vi "Parse TMC_Telemetry.vi"(10 "Variant":variant) -> (2 "Automated_Telemetry":T1 {"Register 1"."Spare" format="%04x"; "Register 2"."Spare" format="%04x"; "Register 4"."Spare" format="%04x"; "Register 5"."Spare" format="%04x"; "Register 6"."Spare" format="%04x"; "Register 7"."Spare" format="%04x"; "Register 8"."Spare" format="%04x"; "Register 9"."Spare" format="%.0x"; "Register 9"."A_D_Value" format="%.0x"; "Register D"."Spare" format="%03x"})   [LabVIEW 2019]
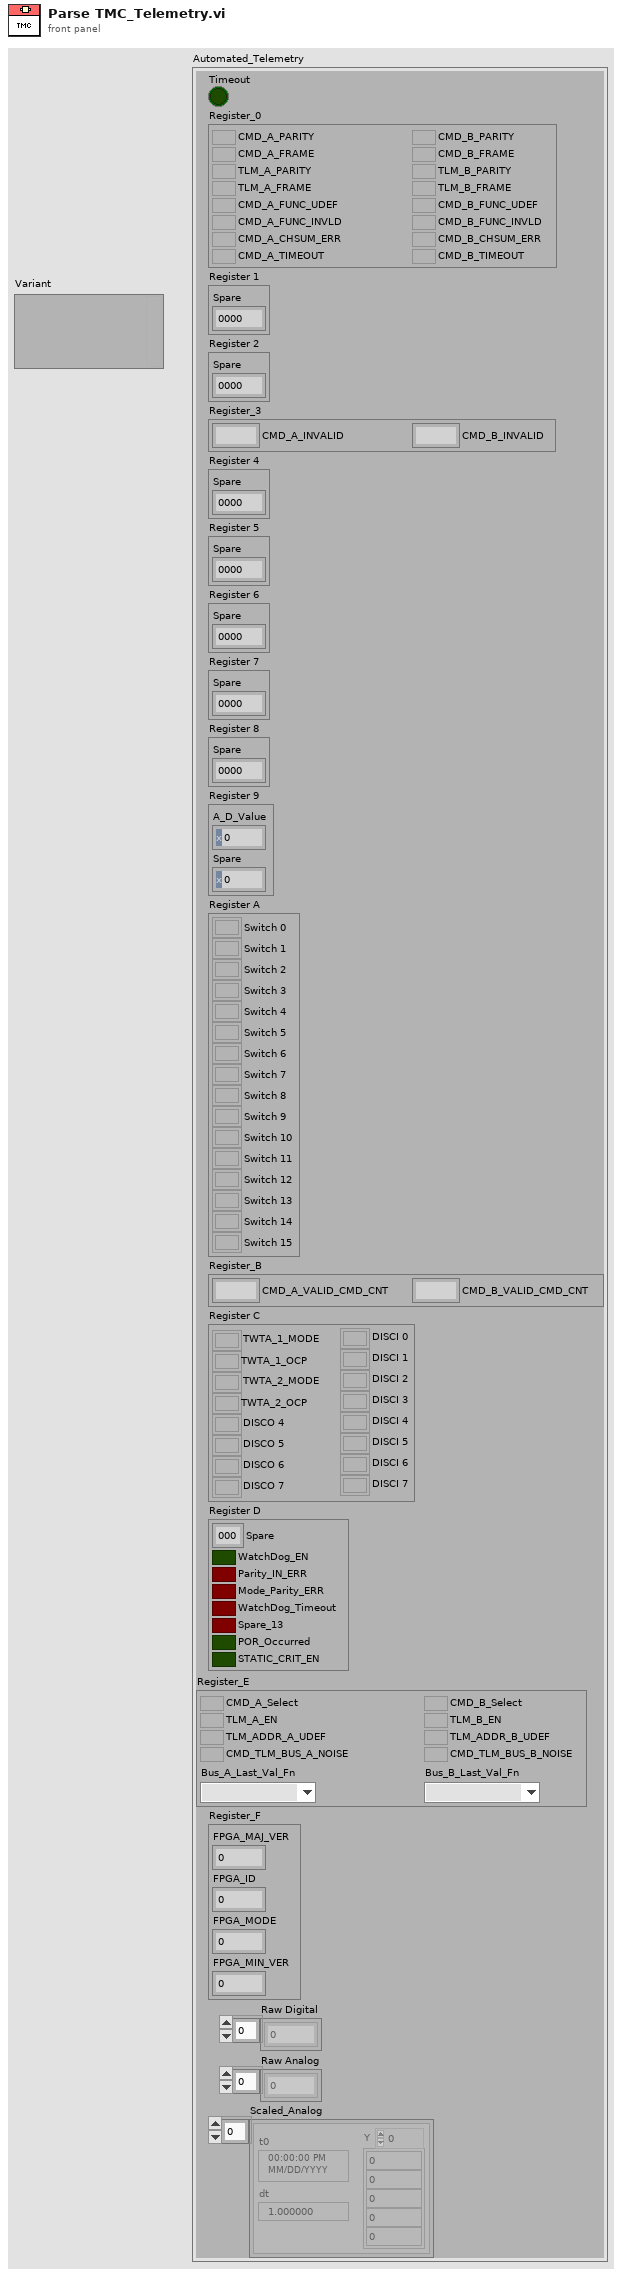
[diagram p1: front panel]
types:
  T1 = cluster{"Timeout":bool, "Register_0":cluster{"CMD_B_PARITY":bool, "CMD_A_PARITY":bool, "CMD_B_FRAME":bool, "CMD_A_FRAME":bool, "TLM_B_PARITY":bool, "TLM_A_PARITY":bool, "TLM_B_FRAME":bool, "TLM_A_FRAME":bool, "CMD_B_FUNC_UDEF":bool, "CMD_A_FUNC_UDEF":bool, "CMD_B_FUNC_INVLD":bool, "CMD_A_FUNC_INVLD":bool, "CMD_B_CHSUM_ERR":bool, "CMD_A_CHSUM_ERR":bool, "CMD_B_TIMEOUT":bool, "CMD_A_TIMEOUT":bool}, "Register 1":cluster{"Spare":u16}, "Register 2":cluster{"Spare":u16}, "Register_3":cluster{"CMD_B_INVALID":u8, "CMD_A_INVALID":u8}, "Register 4":cluster{"Spare":u16}, "Register 5":cluster{"Spare":u16}, "Register 6":cluster{"Spare":u16}, "Register 7":cluster{"Spare":u16}, "Register 8":cluster{"Spare":u16}, "Register 9":cluster{"A_D_Value":u16, "Spare":u8}, "Register A":cluster{"Switch 0":bool, "Switch 1":bool, "Switch 2":bool, "Switch 3":bool, "Switch 4":bool, "Switch 5":bool, "Switch 6":bool, "Switch 7":bool, "Switch 8":bool, "Switch 9":bool, "Switch 10":bool, "Switch 11":bool, "Switch 12":bool, "Switch 13":bool, "Switch 14":bool, "Switch 15":bool}, "Register_B":cluster{"CMD_B_VALID_CMD_CNT":u8, "CMD_A_VALID_CMD_CNT":u8}, "Register C":cluster{"TWTA_1_MODE":bool, "TWTA_1_OCP":bool, "TWTA_2_MODE":bool, "TWTA_2_OCP":bool, "DISCO 4":bool, "DISCO 5":bool, "DISCO 6":bool, "DISCO 7":bool, "DISCI 0":bool, "DISCI 1":bool, "DISCI 2":bool, "DISCI 3":bool, "DISCI 4":bool, "DISCI 5":bool, "DISCI 6":bool, "DISCI 7":bool}, "Register D":cluster{"Spare":u16, "WatchDog_EN":bool, "Parity_IN_ERR":bool, "Mode_Parity_ERR":bool, "WatchDog_Timeout":bool, "Spare_13":bool, "POR_Occurred":bool, "STATIC_CRIT_EN":bool}, "Register_E":cluster{"CMD_B_Select":bool, "CMD_A_Select":bool, "TLM_B_EN":bool, "TLM_A_EN":bool, "TLM_ADDR_B_UDEF":bool, "TLM_ADDR_A_UDEF":bool, "CMD_TLM_BUS_B_NOISE":bool, "CMD_TLM_BUS_A_NOISE":bool, "Bus_B_Last_Val_Fn":enum16{"No_Command", "IO_Comand", "Housekeeping", "Bad_Function"}, "Bus_A_Last_Val_Fn":enum16{"No_Command", "IO_Comand", "Housekeeping", "Bad_Function"}}, "Register_F":cluster{"FPGA_MAJ_VER":u8, "FPGA_ID":u8, "FPGA_MODE":u8, "FPGA_MIN_VER":u8}, "Raw Digital":u16[], "Raw Analog":u16[], "Scaled_Analog":waveform(dbl)[]}
  T2 = cluster{"Timeout":bool, "Register_0":cluster{"CMD_B_PARITY":bool, "CMD_A_PARITY":bool, "CMD_B_FRAME":bool, "CMD_A_FRAME":bool, "TLM_B_PARITY":bool, "TLM_A_PARITY":bool, "TLM_B_FRAME":bool, "TLM_A_FRAME":bool, "CMD_B_FUNC_UDEF":bool, "CMD_A_FUNC_UDEF":bool, "CMD_B_FUNC_INVLD":bool, "CMD_A_FUNC_INVLD":bool, "CMD_B_CHSUM_ERR":bool, "CMD_A_CHSUM_ERR":bool, "CMD_B_TIMEOUT":bool, "CMD_A_TIMEOUT":bool}, "Register 1":cluster{"Spare":u16}, "Register 2":cluster{"Spare":u16}, "Register_3":cluster{"CMD_B_INVALID":u8, "CMD_A_INVALID":u8}, "Register 4":cluster{"Spare":u16}, "Register 5":cluster{"Spare":u16}, "Register 6":cluster{"Spare":u16}, "Register 7":cluster{"Spare":u16}, "Register 8":cluster{"Spare":u16}, "Register 9":cluster{"A_D_Value":u16, "Spare":u8}, "Register A":cluster{"Switch 0":bool, "Switch 1":bool, "Switch 2":bool, "Switch 3":bool, "Switch 4":bool, "Switch 5":bool, "Switch 6":bool, "Switch 7":bool, "Switch 8":bool, "Switch 9":bool, "Switch 10":bool, "Switch 11":bool, "Switch 12":bool, "Switch 13":bool, "Switch 14":bool, "Switch 15":bool}, "Register_B":cluster{"CMD_B_VALID_CMD_CNT":u8, "CMD_A_VALID_CMD_CNT":u8}, "Register C":cluster{"TWTA_1_MODE":bool, "TWTA_1_OCP":bool, "TWTA_2_MODE":bool, "TWTA_2_OCP":bool, "DISCO 4":bool, "DISCO 5":bool, "DISCO 6":bool, "DISCO 7":bool, "DISCI 0":bool, "DISCI 1":bool, "DISCI 2":bool, "DISCI 3":bool, "DISCI 4":bool, "DISCI 5":bool, "DISCI 6":bool, "DISCI 7":bool}, "Register D":cluster{"Spare":u16, "WatchDog_EN":bool, "Parity_IN_ERR":bool, "Mode_Parity_ERR":bool, "WatchDog_Timeout":bool, "Spare":bool, "POR_Occurred":bool, "STATIC_CRIT_EN":bool}, "Register_E":cluster{"CMD_B_Select":bool, "CMD_A_Select":bool, "TLM_B_EN":bool, "TLM_A_EN":bool, "TLM_ADDR_B_UDEF":bool, "TLM_ADDR_A_UDEF":bool, "CMD_TLM_BUS_B_NOISE":bool, "CMD_TLM_BUS_A_NOISE":bool, "Bus_B_Last_Val_Fn":enum16{"No_Command", "IO_Comand", "Housekeeping", "Bad_Function"}, "Bus_A_Last_Val_Fn":enum16{"No_Command", "IO_Comand", "Housekeeping", "Bad_Function"}}, "Register_F":cluster{"FPGA_MAJ_VER":u8, "FPGA_ID":u8, "FPGA_MODE":u8, "FPGA_MIN_VER":u8}, "Raw Digital":u16[], "Raw Analog":u16[], "Scaled_Analog":waveform(dbl)[]}
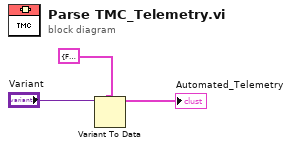
[diagram p0: block diagram]
diagram:
  n1 = Variant To Data(type=T2 {"Timeout"=FALSE, "Register_0"={"CMD_B_PARITY"=FALSE, "CMD_A_PARITY"=FALSE, "CMD_B_FRAME"=FALSE, "CMD_A_FRAME"=FALSE, "TLM_B_PARITY"=FALSE, "TLM_A_PARITY"=FALSE, "TLM_B_FRAME"=FALSE, "TLM_A_FRAME"=FALSE, "CMD_B_FUNC_UDEF"=FALSE, "CMD_A_FUNC_UDEF"=FALSE, "CMD_B_FUNC_INVLD"=FALSE, "CMD_A_FUNC_INVLD"=FALSE, "CMD_B_CHSUM_ERR"=FALSE, "CMD_A_CHSUM_ERR"=FALSE, "CMD_B_TIMEOUT"=FALSE, "CMD_A_TIMEOUT"=FALSE}, "Register 1"={"Spare"=0}, "Register 2"={"Spare"=0}, "Register_3"={"CMD_B_INVALID"=0, "CMD_A_INVALID"=0}, "Register 4"={"Spare"=0}, "Register 5"={"Spare"=0}, "Register 6"={"Spare"=0}, "Register 7"={"Spare"=0}, "Register 8"={"Spare"=0}, "Register 9"={"A_D_Value"=0, "Spare"=0}, "Register A"={"Switch 0"=FALSE, "Switch 1"=FALSE, "Switch 2"=FALSE, "Switch 3"=FALSE, "Switch 4"=FALSE, "Switch 5"=FALSE, "Switch 6"=FALSE, "Switch 7"=FALSE, "Switch 8"=FALSE, "Switch 9"=FALSE, "Switch 10"=FALSE, "Switch 11"=FALSE, "Switch 12"=FALSE, "Switch 13"=FALSE, "Switch 14"=FALSE, "Switch 15"=FALSE}, "Register_B"={"CMD_B_VALID_CMD_CNT"=0, "CMD_A_VALID_CMD_CNT"=0}, "Register C"={"TWTA_1_MODE"=FALSE, "TWTA_1_OCP"=FALSE, "TWTA_2_MODE"=FALSE, "TWTA_2_OCP"=FALSE, "DISCO 4"=FALSE, "DISCO 5"=FALSE, "DISCO 6"=FALSE, "DISCO 7"=FALSE, "DISCI 0"=FALSE, "DISCI 1"=FALSE, "DISCI 2"=FALSE, "DISCI 3"=FALSE, "DISCI 4"=FALSE, "DISCI 5"=FALSE, "DISCI 6"=FALSE, "DISCI 7"=FALSE}, "Register D"={"Spare"=0, "WatchDog_EN"=FALSE, "Parity_IN_ERR"=FALSE, "Mode_Parity_ERR"=FALSE, "WatchDog_Timeout"=FALSE, "Spare"=FALSE, "POR_Occurred"=FALSE, "STATIC_CRIT_EN"=FALSE}, "Register_E"={"CMD_B_Select"=FALSE, "CMD_A_Select"=FALSE, "TLM_B_EN"=FALSE, "TLM_A_EN"=FALSE, "TLM_ADDR_B_UDEF"=FALSE, "TLM_ADDR_A_UDEF"=FALSE, "CMD_TLM_BUS_B_NOISE"=FALSE, "CMD_TLM_BUS_A_NOISE"=FALSE, "Bus_B_Last_Val_Fn"=enum."No_Command", "Bus_A_Last_Val_Fn"=enum."No_Command"}, "Register_F"={"FPGA_MAJ_VER"=0, "FPGA_ID"=0, "FPGA_MODE"=0, "FPGA_MIN_VER"=0}, "Raw Digital"=[], "Raw Analog"=[], "Scaled_Analog"=[]} ("Automated_Telemetry 2"), Variant="Variant") -> (data=→"Automated_Telemetry":T2)  [unwired: 1 in, 1 out]
